vi "Adquirir Parametro Inversor por SNMP.vi"(0 "queue in":refnum<queue>, 7 "error in":errorcluster) -> (13 "result":dbl[](array[numeric]), 14 "Flujo_Bypass":bool, 15 "Time inversor":timestamp, 16 "Flujo_Bat_Carga":bool, 17 "Flujo_Bat_Descarga":bool, 18 "Flujo_Panel":bool, 19 "Flujo_Load":bool, 20 "Pot_Panel_Out":dbl, 21 "Pot_Load_Out":dbl, 22 "Nivel_bat_Out":dbl, 23 "Ring_Panel_Out":i32, 24 "error de conexion":bool, 25 "Ring_Nivel_Bat_Out":i32, 26 "Ring_Inversor_Out":i32, 27 "error out":errorcluster)   [LabVIEW 2015]
uses:
  Application/ClusterM2.ctl
  Login Window Control Folder/global variable.vi
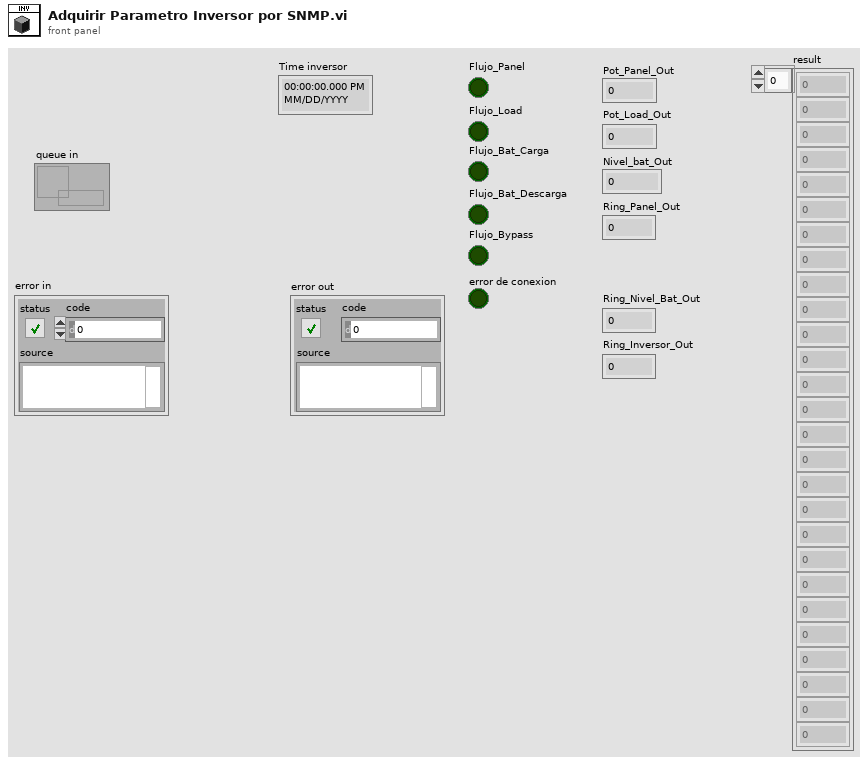
[diagram p1: front panel]
types:
  T1 = typedef "ClusterM2.ctl" = cluster{"timeStamp":timestamp, "Data":dbl[], "group":string}
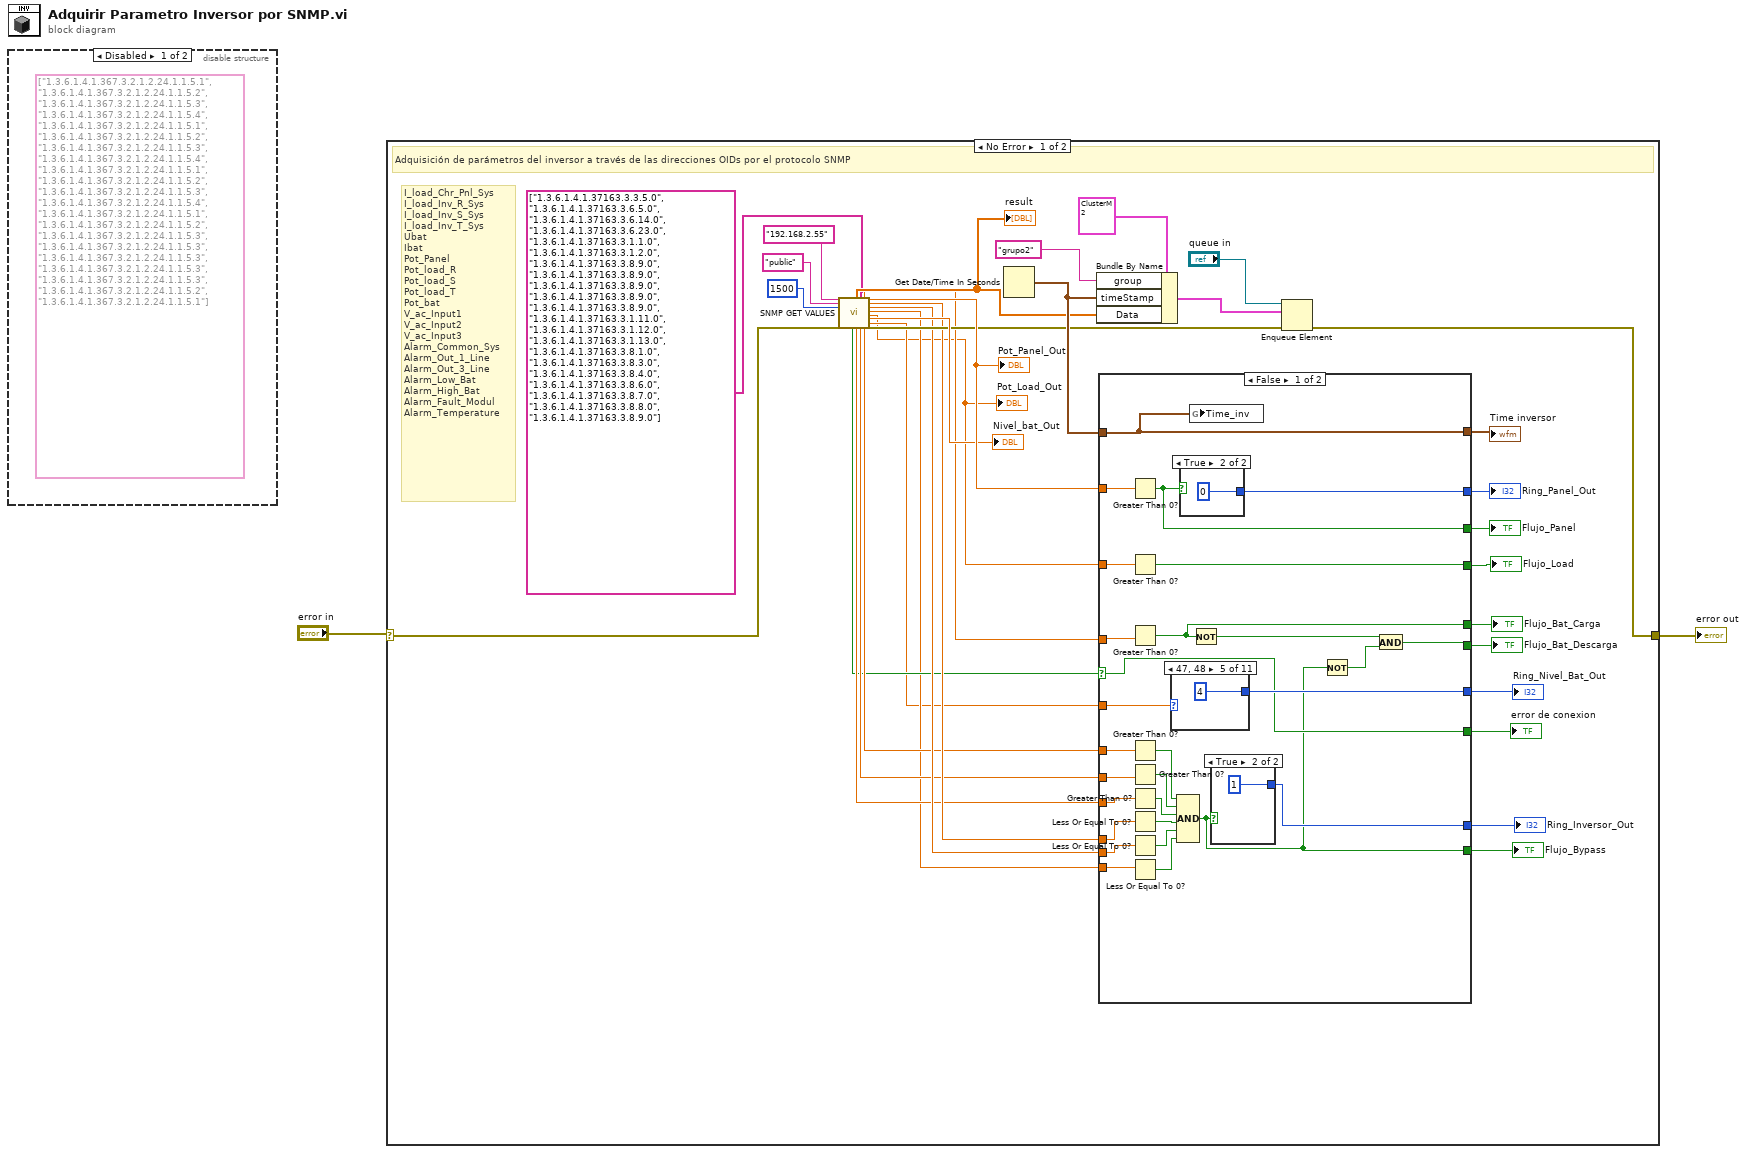
[diagram p0: block diagram]
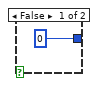
[diagram p3: hidden frame]
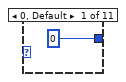
[diagram p4: hidden frame]
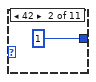
[diagram p5: hidden frame]
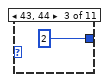
[diagram p6: hidden frame]
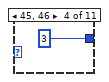
[diagram p7: hidden frame]
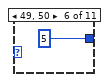
[diagram p8: hidden frame]
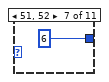
[diagram p9: hidden frame]
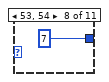
[diagram p10: hidden frame]
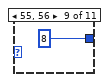
[diagram p11: hidden frame]
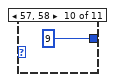
[diagram p12: hidden frame]
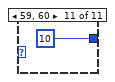
[diagram p13: hidden frame]
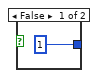
[diagram p14: hidden frame]
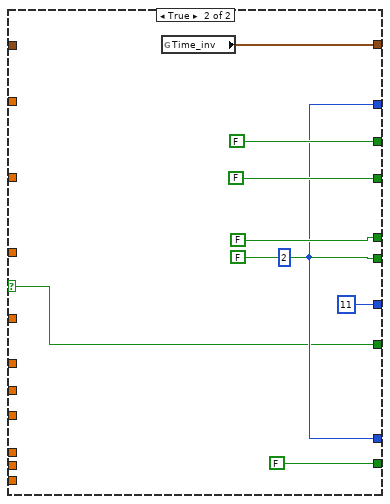
[diagram p15: hidden frame]
diagram:
  n1 = disable-structure shown="Disabled" {
    frame Disabled {
      (unwired) string[] ["1.3.6.1.4.1.367.3.2.1.2.24.1.1.5.1", "1.3.6.1.4.1.367.3.2.1.2.24.1.1.5.2", "1.3.6.1.4.1.367.3.2.1.2.24.1.1.5.3", "1.3.6.1.4.1.367.3.2.1.2.24.1.1.5.4", "1.3.6.1.4.1.367.3.2.1.2.24.1.1.5.1", "1.3.6.1.4.1.367.3.2.1.2.24.1.1.5.2", "1.3.6.1.4.1.367.3.2.1.2.24.1.1.5.3", "1.3.6.1.4.1.367.3.2.1.2.24.1.1.5.4", "1.3.6.1.4.1.367.3.2.1.2.24.1.1.5.1", "1.3.6.1.4.1.367.3.2.1.2.24.1.1.5.2", "1.3.6.1.4.1.367.3.2.1.2.24.1.1.5.3", "1.3.6.1.4.1.367.3.2.1.2.24.1.1.5.4", "1.3.6.1.4.1.367.3.2.1.2.24.1.1.5.1", "1.3.6.1.4.1.367.3.2.1.2.24.1.1.5.2", "1.3.6.1.4.1.367.3.2.1.2.24.1.1.5.3", "1.3.6.1.4.1.367.3.2.1.2.24.1.1.5.3", "1.3.6.1.4.1.367.3.2.1.2.24.1.1.5.3", "1.3.6.1.4.1.367.3.2.1.2.24.1.1.5.3", "1.3.6.1.4.1.367.3.2.1.2.24.1.1.5.3", "1.3.6.1.4.1.367.3.2.1.2.24.1.1.5.2", "1.3.6.1.4.1.367.3.2.1.2.24.1.1.5.1"]
    }
    frame Enabled {
    }
  }
  n2 = case shown="No Error" "error in" {
    selector: "error in" -> [w11 w90]
    tunnel: [w10 w90] -> w2
    frame No Error {
      # "I_load_Chr_Pnl_Sys\nI_load_Inv_R_Sys\nI_load_Inv_S_Sys\nI_load_Inv_T_Sys\nUbat\nIbat\nPot_Panel\nPot_load_R\nPot_load_S\nPot_load_T\nPot_bat\nV_ac_Input1\nV_ac_Input2\nV_ac_Input3\nAlarm_Common_Sys\nAlarm_Out_1_Line\nAlarm_Out_3_Line\nAlarm_Low_Bat\nAlarm_High_Bat\nAlarm_Fault_Modul\nAlarm_Temperature"
      # "Adquisición de parámetros del inversor a través de las direcciones OIDs por el protocolo SNMP"
      n3 = call "SNMP GET VALUES.vi"("IP Address"="192.168.2.55", "Community"="public", "Timeout"=1500, "error in"=w11, "OIDs"=string[] ["1.3.6.1.4.1.37163.3.3.5.0", "1.3.6.1.4.1.37163.3.6.5.0", "1.3.6.1.4.1.37163.3.6.14.0", "1.3.6.1.4.1.37163.3.6.23.0", "1.3.6.1.4.1.37163.3.1.1.0", "1.3.6.1.4.1.37163.3.1.2.0", "1.3.6.1.4.1.37163.3.8.9.0", "1.3.6.1.4.1.37163.3.8.9.0", "1.3.6.1.4.1.37163.3.8.9.0", "1.3.6.1.4.1.37163.3.8.9.0", "1.3.6.1.4.1.37163.3.8.9.0", "1.3.6.1.4.1.37163.3.1.11.0", "1.3.6.1.4.1.37163.3.1.12.0", "1.3.6.1.4.1.37163.3.1.13.0", "1.3.6.1.4.1.37163.3.8.1.0", "1.3.6.1.4.1.37163.3.8.3.0", "1.3.6.1.4.1.37163.3.8.4.0", "1.3.6.1.4.1.37163.3.8.6.0", "1.3.6.1.4.1.37163.3.8.7.0", "1.3.6.1.4.1.37163.3.8.8.0", "1.3.6.1.4.1.37163.3.8.9.0"]) -> ("error snmp"=w12:bool, "result"=w9:dbl[], "Vac_input3"=w13:dbl, "Vac_input2"=w14:dbl, "Ibat"=w5:dbl, "Vac_input1"=w15:dbl, "Pot_panel_out"=w22:dbl, "I_Load_Inv_R"=w19:dbl, "I_Load_Inv_S"=w18:dbl, "I_Load_Inv_T"=w7:dbl, "Pot_load_out"=w4:dbl, "Nivel_bat_out"=→"Nivel_bat_Out":dbl, "Ubat"=w6:dbl, "error out"=w20:errorcluster)  [unwired: 9 in]
      "Pot_Load_Out" <- w4
      "Pot_Panel_Out" <- w22
      "result" <- w9
      n4 = Get Date/Time In Seconds() -> (seconds since 1Jan1904=w33:timestamp)
      n5 = Bundle By Name(cluster=T1 {"timeStamp"=timestamp(0 s since 1904-01-01), "Data"=[], "group"=""} ("M2"), "group"="grupo2", "timeStamp"=w33, "Data"=w9) -> (w36:T1)
      n6 = case shown="False" w12 {
        selector: w12 -> [w42 w81]
        tunnel: w33 -> [w65 _]
        tunnel: w22 -> [w45 _]
        tunnel: w4 -> [w46 _]
        tunnel: w5 -> [w48 _]
        tunnel: [w65 w89] -> w32
        tunnel: [w64 w83] -> w31
        tunnel: [w44 FALSE] -> w30
        tunnel: [w43 FALSE] -> w29
        tunnel: [w47 FALSE] -> w28
        tunnel: [w40 FALSE] -> w27
        tunnel: w6 -> [w63 _]
        tunnel: [w62 11] -> w26
        tunnel: w15 -> [w61 _]
        tunnel: w14 -> [w60 _]
        tunnel: w13 -> [w59 _]
        tunnel: w19 -> [w58 _]
        tunnel: w18 -> [w56 _]
        tunnel: w7 -> [w57 _]
        tunnel: [w38 FALSE] -> w17
        tunnel: [w55 w83] -> w16
        tunnel: [w42 w81] -> w3
        frame False {
          n7 = Greater Than 0?(x=w45) -> (x > 0?=w44:bool)
          n8 = Greater Than 0?(x=w46) -> (x > 0?=w43:bool)
          n9 = Greater Than 0?(x=w48) -> (x > 0?=w47:bool)
          n10 = Greater Than 0?(x=w61) -> (x > 0?=w54:bool)
          n11 = Greater Than 0?(x=w60) -> (x > 0?=w53:bool)
          n12 = Greater Than 0?(x=w59) -> (x > 0?=w52:bool)
          n13 = Less Or Equal To 0?(x=w58) -> (x <= 0?=w51:bool)
          n14 = Less Or Equal To 0?(x=w56) -> (x <= 0?=w50:bool)
          n15 = Less Or Equal To 0?(x=w57) -> (x <= 0?=w49:bool)
          n16 = case shown="47, 48" w63 {
            tunnel: [0 1 2 3 4 5 6 7 8 9 10] -> w62
            frame 0, Default {
            }
            frame 42 {
            }
            frame 43, 44 {
            }
            frame 45, 46 {
            }
            frame 47, 48 {
            }
            frame 49, 50 {
            }
            frame 51, 52 {
            }
            frame 53, 54 {
            }
            frame 55, 56 {
            }
            frame 57, 58 {
            }
            frame 59, 60 {
            }
          }
          n17 = Compound Arithmetic op=AND(w54, w53, w52, w51, w50, w49) -> (w38:bool)
          n18 = case shown="True" w44 {
            tunnel: [1 0] -> w64
            frame False {
            }
            frame True {
            }
          }
          n19 = global write "global variable.vi" "Time_inv"(w65) -> ()
          n20 = Not(x=w47) -> (.not. x?=w41:bool)
          n21 = case shown="True" w38 {
            tunnel: [0 1] -> w55
            frame False {
            }
            frame True {
            }
          }
          n22 = Not(x=w38) -> (.not. x?=w39:bool)
          n23 = And(x=w41, y=w39) -> (x .and. y?=w40:bool)
        }
        frame True {
          w83 = 2
          n24 = global read "global variable.vi" "Time_inv"() -> (w89:timestamp)
        }
      }
      "Time inversor" <- w32
      "Ring_Panel_Out" <- w31
      "Ring_Nivel_Bat_Out" <- w26
      "Flujo_Panel" <- w30
      "Flujo_Load" <- w29
      "Flujo_Bat_Carga" <- w28
      "Flujo_Bat_Descarga" <- w27
      "Flujo_Bypass" <- w17
      "Ring_Inversor_Out" <- w16
      "error de conexion" <- w3
      n25 = Enqueue Element(queue="queue in", element=w36, error in (no error)=w20) -> (error out=w10:errorcluster)  [unwired: 1 in, 2 out]
    }
    frame Error {
    }
  }
  "error out" <- w2
